vi "RunMeas.vi"(8 "error in (no error)":errorcluster, 11 "PacificPowerSource in":refnum<class "PacificPowerSource.lvclass">) -> (0 "error out":errorcluster, 3 "PacificPowerSource out":refnum<class "PacificPowerSource.lvclass">)   [LabVIEW 2018, in "AcPwrPlugins.lvlib" / "PacificPowerSource.lvclass"]
doc: "This VI (may) start and retrieve measurements from the instruments."
uses:
  PacificPowerSource.lvclass
  C:/Users/ico/Documents/Projects/NistPluggableModules/AcPwr/AcPwrPlugins/AcPwrBaseClass/AcPwrBase.lvclass
  AcPwrBaseClass/AcPwrBase.lvclass/AcPwrBase.ctl
  AcPwrBaseClass/Accessors/Read RefreshTime.vi
  <instrlib>/Pacific Power UPC Series/Public/Data/Read (Single).vi
  <instrlib>/Pacific Power UPC Series/Pacific Power UPC Series.lvlib
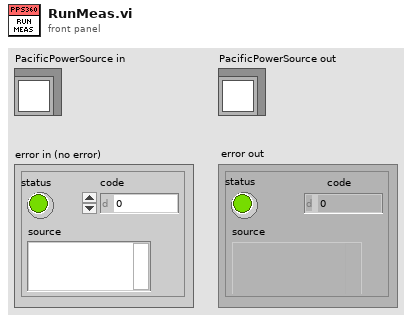
[diagram p1: front panel]
types:
  T1 = typedef "AcPwrPlugins.lvlib/PacificPowerSource.lvclass/Measurements.ctl" = cluster{"Handle":string, "Name":string, "Enabled":bool, "Measurement Value":dbl, "Channel Name(1: A)":u16, "Measurement Type (0: Voltage RMS L-N)":u16}[]
  T2 = cluster{"Handle":string, "Name":string, "Enabled":bool, "Measurement Value":dbl, "Channel Name(1: A)":u16, "Measurement Type (0: Voltage RMS L-N)":u16}
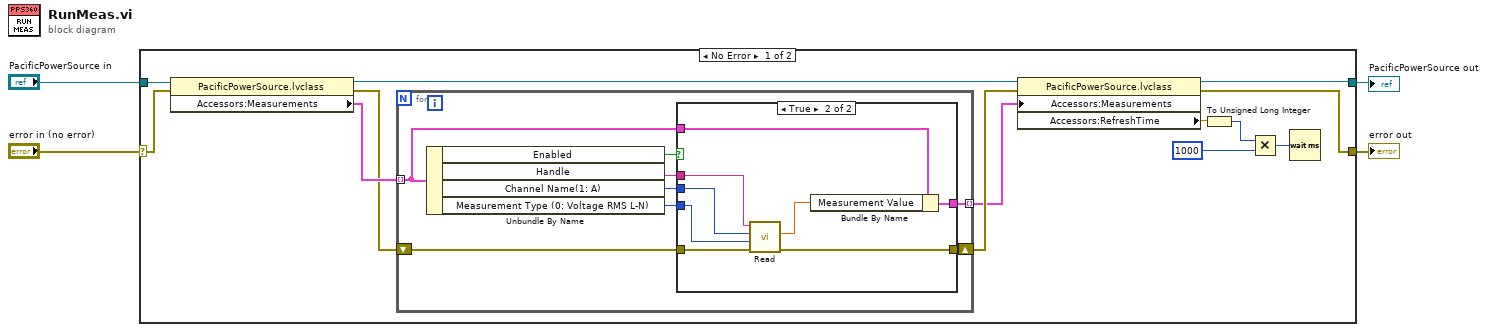
[diagram p0: block diagram]
diagram:
  n1 = case shown="No Error" "error in (no error)" {
    selector: "error in (no error)" -> [w16 w36]
    tunnel: [w10 w36] -> w1
    tunnel: [w11 w37] -> w2
    tunnel: "PacificPowerSource in" -> [w17 w37]
    frame No Error {
      n2 = property class="PacificPowerSource.lvclass"(reference=w17, error in=w16) -> (reference out=w13:refnum<class "PacificPowerSource.lvclass">, error out=w14:errorcluster, "Accessors:Measurements"=w15:T1)
      n3 = for {
        tunnel: w15 -> [w25] mode=indexing
        tunnel: [w24] -> w9 mode=indexing
        shift-right: [w21] -> w12
        shift-left: w14 -> [w23]
        n4 = Unbundle By Name(w25) -> ("Enabled"=w20:bool, "Handle"=w22:string, "Channel Name(1: A)"=w19:u16, "Measurement Type (0: Voltage RMS L-N)"=w18:u16)
        n5 = case shown="True" w20 {
          tunnel: w25 -> [w26 w35]
          tunnel: [w26 w34] -> w24
          tunnel: w23 -> [w27 w31]
          tunnel: w22 -> [_ w28]
          tunnel: [w27 w32] -> w21
          tunnel: w19 -> [_ w30]
          tunnel: w18 -> [_ w29]
          frame False {
          }
          frame True {
            n6 = call-poly <instrlib>:"Read.vi"("error in (no error)"=w31, "Measurement Type (0: Voltage RMS L-N)"=w29, "Channel Name(1: A)"=w30, "VISA resource name"=w28) -> ("error out"=w32:errorcluster, "Measurement"=w33:dbl)  [unwired: 5 in, 1 out]
            n7 = Bundle By Name(cluster=w35, "Measurement Value"=w33) -> (w34:T2)
          }
        }
      }
      n8 = property class="PacificPowerSource.lvclass"(reference=w13, error in=w12, "Accessors:Measurements"=w9) -> (reference out=w11:refnum<class "PacificPowerSource.lvclass">, error out=w10:errorcluster, "Accessors:RefreshTime"=w6:dbl)
      n9 = To Unsigned Long Integer(number=w6) -> (unsigned 32bit integer=w5:u32)
      n10 = Multiply(x=w5, y=u32 1000) -> (x*y=w7:u32)
      n11 = Wait (ms)(milliseconds to wait=w7) -> ()  [unwired: 1 out]
    }
    frame Error {
    }
  }
  "PacificPowerSource out" <- w2
  "error out" <- w1
